vi "ex_6.vi"() -> ()   [LabVIEW 2020]
uses:
  #typedef_Product.ctl
  #typedef_Enum_sort.ctl
  #typedef_SM_States.ctl
  #typedef_ProgramData.ctl
panel:
  in  "Sort by":T1
  in  "Sort":bool
  in  "Product Number, Name or Producer":string
  in  "Search Product":bool
  in  "Save to file":bool
  in  "Read from file":bool
  in  "Previous":bool
  in  "Next":bool
  out "Product":T2
  in  "Stop Program":bool
  in  "Remove Product":bool
  in  "Add Product":bool
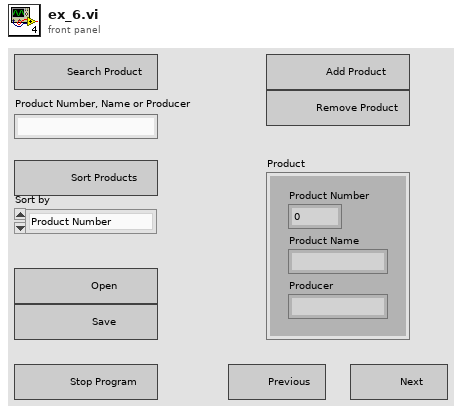
[diagram p1: front panel]
types:
  T1 = typedef "#typedef_Enum_sort.ctl" = enum16{"Product Number", "Product Name", "Producer"}
  T2 = typedef "#typedef_Product.ctl" = cluster{"Product Number":i32, "Product Name":string, "Producer":string}
  T3 = typedef "#typedef_SM_States.ctl" = enum16{"Initialize", "Idle", "Add Product", "Remove Product", "Show Next", "Show Previous", "RefreshGUI", "Save", "Read", "Search", "Sort", "Error Handler", "Save Before Exit", "Exit"}
  T4 = typedef "#typedef_ProgramData.ctl" = cluster{"Products":T2[], "Current Product":i32, "Product Data":path, "Search Number, Name or Producer":string, "Sort by":T1}
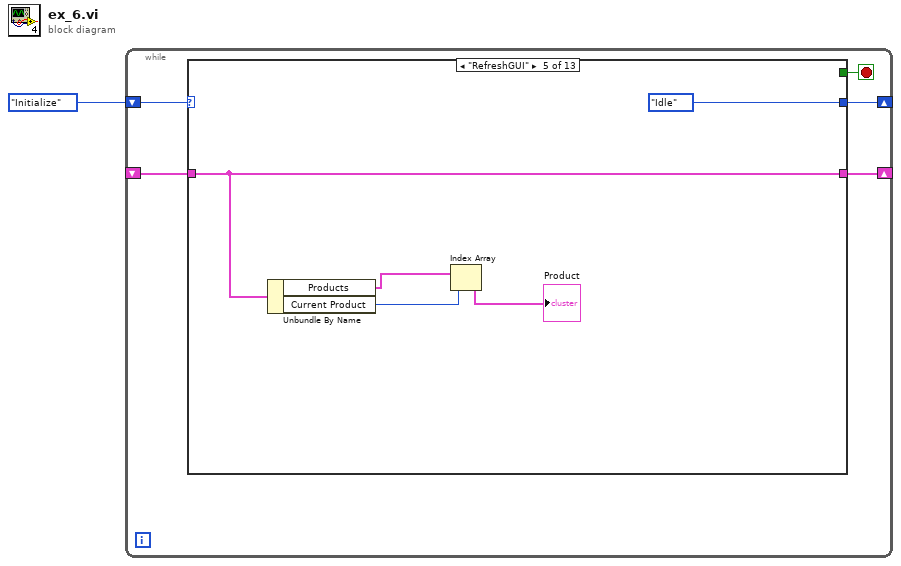
[diagram p0: block diagram]
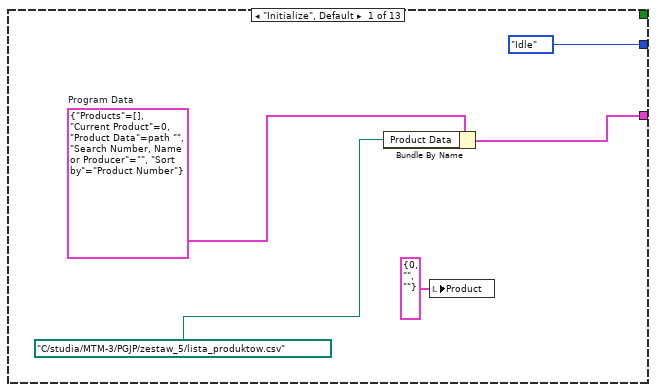
[diagram p2: hidden frame]
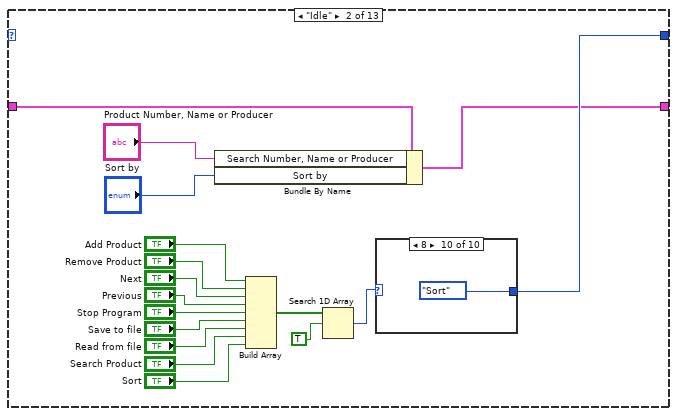
[diagram p3: hidden frame]
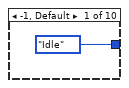
[diagram p4: hidden frame]
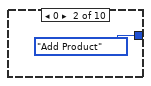
[diagram p5: hidden frame]
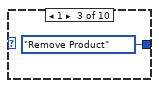
[diagram p6: hidden frame]
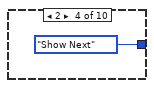
[diagram p7: hidden frame]
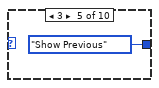
[diagram p8: hidden frame]
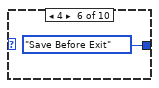
[diagram p9: hidden frame]
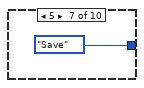
[diagram p10: hidden frame]
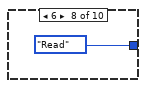
[diagram p11: hidden frame]
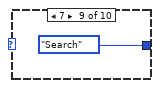
[diagram p12: hidden frame]
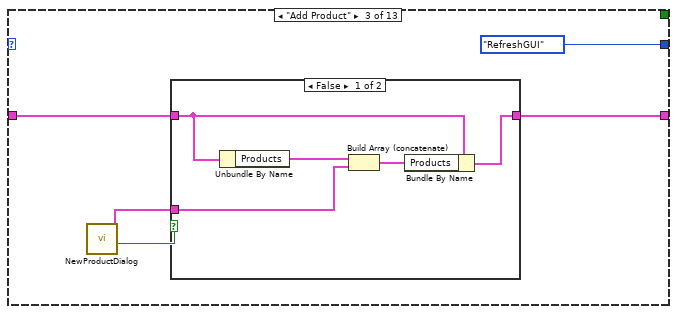
[diagram p13: hidden frame]
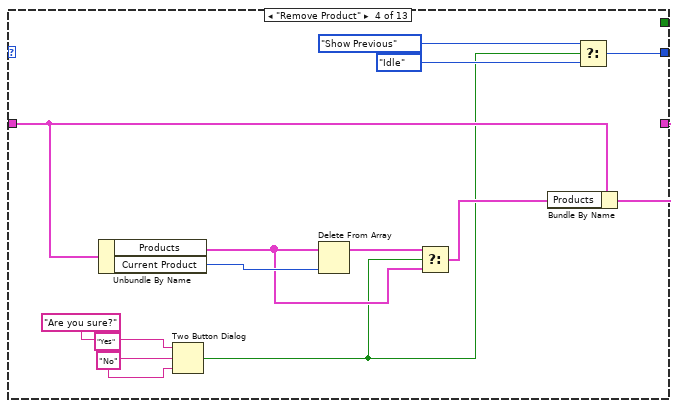
[diagram p15: hidden frame]
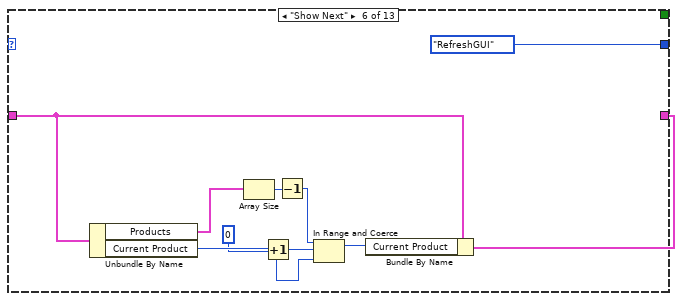
[diagram p16: hidden frame]
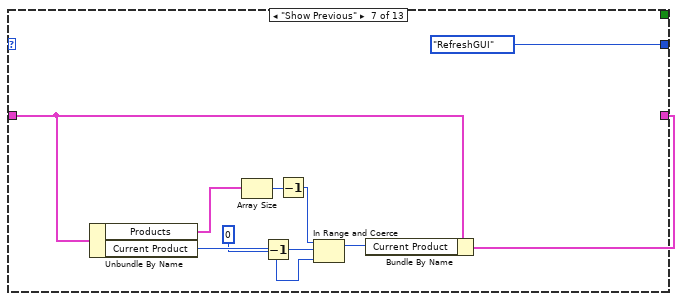
[diagram p17: hidden frame]
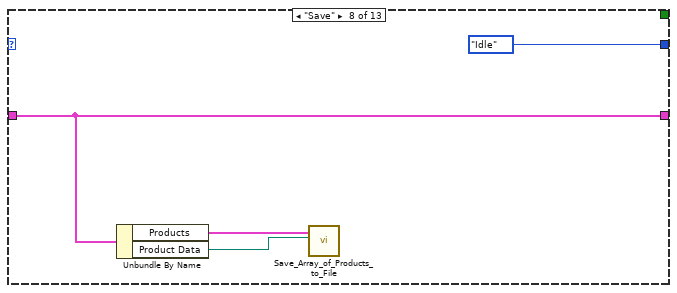
[diagram p18: hidden frame]
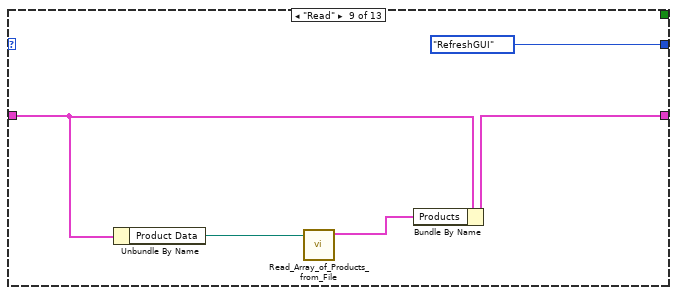
[diagram p19: hidden frame]
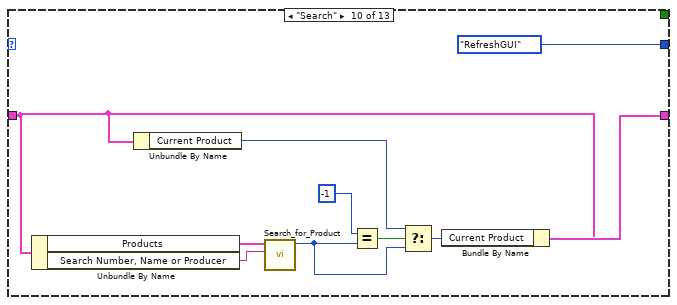
[diagram p20: hidden frame]
diagram:
  n1 = while {
    shift-right: [w4] -> _
    shift-left: #typedef_SM_States."Initialize" ("SM_States") -> [w6]
    shift-right: [w3] -> _
    shift-left: _ -> [w2]
    stop <- w5 stop-if-true
    n2 = case shown="\"RefreshGUI\"" w6 {
      tunnel: [_ _ _ _ _ _ _ _ _ _ _ _ TRUE] -> w5
      tunnel: [#typedef_SM_States."Idle" ("SM_States") w20 #typedef_SM_States."RefreshGUI" ("SM_States") w50 #typedef_SM_States."Idle" ("SM_States") #typedef_SM_States."RefreshGUI" ("SM_States") #typedef_SM_States."RefreshGUI" ("SM_States") #typedef_SM_States."Idle" ("SM_States") #typedef_SM_States."RefreshGUI" ("SM_States") #typedef_SM_States."RefreshGUI" ("SM_States") #typedef_SM_States."RefreshGUI" ("SM_States") #typedef_SM_States."Exit" ("SM_States") #typedef_SM_States."Exit" ("SM_States")] -> w4
      tunnel: [w9 w15 w41 w62 w67 w74 w84 w91 w95 w103 w108 w143 w144] -> w3
      tunnel: w2 -> [_ w16 w40 w55 w67 w76 w86 w91 w94 w102 w109 w143 w144]
      frame "Initialize", Default {
        w10 = T4 {"Products"=[], "Current Product"=0, "Product Data"=path "", "Search Number, Name or Producer"="", "Sort by"=enum."Product Number"}  # Program Data
        n3 = Bundle By Name(cluster=w10, "Product Data"=path "C:/studia/MTM-3/PGJP/zestaw_5/lista_produktow.csv") -> (w9:T4)
        n4 = local write "Product"(T2 {"Product Number"=0, "Product Name"="", "Producer"=""} ("Product")) -> ()
      }
      frame "Idle" {
        n5 = Bundle By Name(cluster=w16, "Search Number, Name or Producer"="Product Number, Name or Producer", "Sort by"="Sort by") -> (w15:T4)
        n6 = Build Array("Add Product", "Remove Product", "Next", "Previous", "Stop Program", "Save to file", "Read from file", "Search Product", "Sort") -> (w23:bool[])
        n7 = Search 1D Array(1D array=w23, element=TRUE) -> (index of element=w21:i32)  [unwired: 1 in]
        n8 = case shown="8" w21 {
          tunnel: [#typedef_SM_States."Idle" ("SM_States") #typedef_SM_States."Add Product" ("SM_States") #typedef_SM_States."Remove Product" ("SM_States") #typedef_SM_States."Show Next" ("SM_States") #typedef_SM_States."Show Previous" ("SM_States") #typedef_SM_States."Save Before Exit" ("SM_States") #typedef_SM_States."Save" ("SM_States") #typedef_SM_States."Read" ("SM_States") #typedef_SM_States."Search" ("SM_States") #typedef_SM_States."Sort" ("SM_States")] -> w20
          frame -1, Default {
          }
          frame 0 {
          }
          frame 1 {
          }
          frame 2 {
          }
          frame 3 {
          }
          frame 4 {
          }
          frame 5 {
          }
          frame 6 {
          }
          frame 7 {
          }
          frame 8 {
          }
        }
      }
      frame "Add Product" {
        n9 = call "NewProductDialog.vi"() -> ("Cancelled?"=w39:bool, "New Product"=w42:T2)  [unwired: 9 in, 1 out]
        n10 = case shown="False" w39 {
          tunnel: w42 -> [w48 _]
          tunnel: [w47 w49] -> w41
          tunnel: w40 -> [w45 w49]
          frame False {
            n11 = Unbundle By Name(w45) -> ("Products"=w46:T2[])
            n12 = Build Array (concatenate)(w46, w48) -> (w44:T2[])
            n13 = Bundle By Name(cluster=w45, "Products"=w44) -> (w47:T4)
          }
          frame True {
          }
        }
      }
      frame "Remove Product" {
        n14 = Unbundle By Name(w55) -> ("Products"=w54:T2[], "Current Product"=w61:i32)
        n15 = Two Button Dialog(message="Are you sure?", 1:"No" ("F button name (\"Cancel\")"), 2:"Yes" ("button name (\"OK\")")) -> (T button?=w51:bool)
        n16 = Delete From Array(array=w54, index=w61) -> (array with subset deleted=w56:T2[])  [unwired: 1 in, 1 out]
        n17 = Select(t=w56, s=w51, f=w54) -> (s? t:f=w57:T2[])
        n18 = Bundle By Name(cluster=w55, "Products"=w57) -> (w62:T4)
        n19 = Select(t=#typedef_SM_States."Show Previous" ("SM_States"), s=w51, f=#typedef_SM_States."Idle" ("SM_States")) -> (s? t:f=w50:T3)
      }
      frame "RefreshGUI" {
        n20 = Unbundle By Name(w67) -> ("Products"=w66:T2[], "Current Product"=w63:i32)
        n21 = Index Array(array=w66, index=w63) -> (element=→"Product":T2)
      }
      frame "Show Next" {
        n22 = Unbundle By Name(w76) -> ("Products"=w73:T2[], "Current Product"=w75:i32)
        n23 = Array Size(array=w73) -> (size(s)=w70:i32)
        n24 = Increment(x=w75) -> (x+1=w72:i32)
        n25 = Decrement(x=w70) -> (x-1=w68:i32)
        n26 = In Range and Coerce(upper limit=w68, x=w72, lower limit=0) -> (coerced(x)=w69:i32)  [unwired: 1 out]
        n27 = Bundle By Name(cluster=w76, "Current Product"=w69) -> (w74:T4)
      }
      frame "Show Previous" {
        n28 = Unbundle By Name(w86) -> ("Products"=w83:T2[], "Current Product"=w85:i32)
        n29 = Array Size(array=w83) -> (size(s)=w80:i32)
        n30 = Decrement(x=w85) -> (x-1=w82:i32)
        n31 = Decrement(x=w80) -> (x-1=w78:i32)
        n32 = In Range and Coerce(upper limit=w78, x=w82, lower limit=0) -> (coerced(x)=w79:i32)  [unwired: 1 out]
        n33 = Bundle By Name(cluster=w86, "Current Product"=w79) -> (w84:T4)
      }
      frame "Save" {
        n34 = Unbundle By Name(w91) -> ("Products"=w90:T2[], "Product Data"=w88:path)
        n35 = call "Save_Array_of_Products_to_File.vi"("Path"=w88, "array of #typedef Products"=w90) -> ()  [unwired: 10 in]
      }
      frame "Read" {
        n36 = Unbundle By Name(w94) -> ("Product Data"=w93:path)
        n37 = call "Read_Array_of_Products_from_File.vi"("Path"=w93) -> ("Array"=w92:T2[])  [unwired: 10 in]
        n38 = Bundle By Name(cluster=w94, "Products"=w92) -> (w95:T4)
      }
      frame "Search" {
        n39 = Unbundle By Name(w102) -> ("Products"=w105:T2[], "Search Number, Name or Producer"=w104:string)
        n40 = Unbundle By Name(w102) -> ("Current Product"=w100:i32)
        n41 = call "Search_for_Product.vi"("Search Number, Name or Producer"=w104, "Products"=w105) -> ("Product Index"=w97:i32)  [unwired: 8 in, 1 out]
        n42 = Equal?(x=-1 ("y"), y=w97) -> (x = y?=w101:bool)
        n43 = Select(t=w100, s=w101, f=w97) -> (s? t:f=w99:i32)
        n44 = Bundle By Name(cluster=w102, "Current Product"=w99) -> (w103:T4)
      }
      frame "Sort" {
        n45 = Unbundle By Name(w109) -> ("Products"=w110:T2[], "Sort by"=w111:T1)
        n46 = case shown="\"Product Name\"" w111 {
          tunnel: w110 -> [w116 w125 w134]
          tunnel: [w113 w122 w131] -> w107
          frame "Product Number" {
            n47 = for {
              tunnel: w116 -> [w121] mode=indexing
              tunnel: [w119] -> w115 mode=indexing
              n48 = Unbundle By Name(w121) -> ("Product Number"=w120:i32)
              n49 = Bundle("Product Number"=w120, "Product"=w121) -> (w119:cluster{"Product Number":i32, "Product":T2})  [unwired: 1 in]
            }
            n50 = Sort 1D Array(array=w115) -> (sorted array=w114:cluster{"Product Number":i32, "Product":T2}[])
            n51 = for {
              tunnel: w114 -> [w118] mode=indexing
              tunnel: [w117] -> w113 mode=indexing
              n52 = Unbundle(w118) -> ("Product"=w117:T2)  [unwired: 1 out]
            }
          }
          frame "Product Name" {
            n53 = for {
              tunnel: w125 -> [w130] mode=indexing
              tunnel: [w128] -> w124 mode=indexing
              n54 = Unbundle By Name(w130) -> ("Product Name"=w129:string)
              n55 = Bundle("Product Name"=w129, "Product"=w130) -> (w128:cluster{"Product Name":string, "Product":T2})  [unwired: 1 in]
            }
            n56 = Sort 1D Array(array=w124) -> (sorted array=w123:cluster{"Product Name":string, "Product":T2}[])
            n57 = for {
              tunnel: w123 -> [w127] mode=indexing
              tunnel: [w126] -> w122 mode=indexing
              n58 = Unbundle(w127) -> ("Product"=w126:T2)  [unwired: 1 out]
            }
          }
          frame "Producer" {
            n59 = for {
              tunnel: w134 -> [w139] mode=indexing
              tunnel: [w137] -> w133 mode=indexing
              n60 = Unbundle By Name(w139) -> ("Producer"=w138:string)
              n61 = Bundle("Producer"=w138, "Product"=w139) -> (w137:cluster{"Producer":string, "Product":T2})  [unwired: 1 in]
            }
            n62 = Sort 1D Array(array=w133) -> (sorted array=w132:cluster{"Producer":string, "Product":T2}[])
            n63 = for {
              tunnel: w132 -> [w136] mode=indexing
              tunnel: [w135] -> w131 mode=indexing
              n64 = Unbundle(w136) -> ("Product"=w135:T2)  [unwired: 1 out]
            }
          }
        }
        n65 = Bundle By Name(cluster=w109, "Products"=w107) -> (w108:T4)
      }
      frame "Save Before Exit" {
        n66 = Unbundle By Name(w143) -> ("Products"=w142:T2[], "Product Data"=w140:path)
        n67 = call "Save_Array_of_Products_to_File.vi"("Path"=w140, "array of #typedef Products"=w142) -> ()  [unwired: 10 in]
      }
      frame "Exit" {
      }
    }
  }
